vi "Map_2Buttons_To_Throttle_Multi_Power.vi"(5 "Power_Down":dbl=1.0, 7 "Power_Up":dbl=1.0, 9 "Down":bool=TRUE, 10 "Up":bool=TRUE) -> (2 "Throttle":dbl)   [LabVIEW 2019]
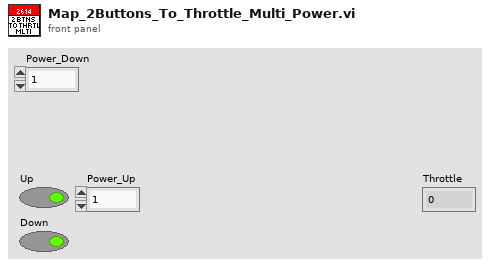
[diagram p1: front panel]
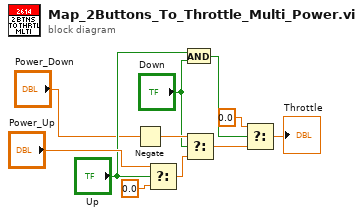
[diagram p0: block diagram]
diagram:
  n1 = Negate(x="Power_Down") -> (-x=w8:dbl)
  n2 = Select(t="Power_Up", s="Up", f=0.0) -> (s? t:f=w10:dbl)
  n3 = And(x="Up", y="Down") -> (x .and. y?=w7:bool)
  n4 = Select(t=w8, s="Down", f=w10) -> (s? t:f=w2:dbl)
  n5 = Select(t=0.0, s=w7, f=w2) -> (s? t:f=→"Throttle":dbl)
